vi "formatCalibratedFieldString.vi"(10 "unit":string="m", 11 "numIn":dbl) -> (3 "formatedNumber":string)   [LabVIEW 2016, in "calibratedIOField.xctl"]
uses:
  calibratedIOField.xctl
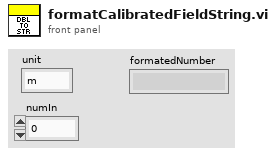
[diagram p1: front panel]
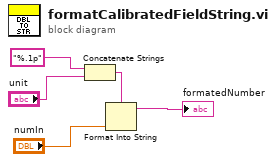
[diagram p0: block diagram]
diagram:
  n1 = Concatenate Strings("%.1p" ("format string"), "unit") -> (w4:string)
  n2 = Format Into String(format string=w4, "numIn") -> (resulting string=→"formatedNumber":string)  [unwired: 2 in, 1 out]
